vi "PAN_RunProc.vi"(0 "Database RefNum in":T1, 1 "module name":string, 7 "VItoRun":string, 11 "error in (no error)":errorcluster, 12 "wait":bool=TRUE) -> (6 "Result":string, 15 "error out":errorcluster)   [LabVIEW 2016]
uses:
  Modules/DBSHAND/private/vis/DatabaseHand_RefNum.ctl
  <vilib>/Utility/error.llb/DialogType.ctl
  Modules/DBSHAND/private/vis/DatabaseHand_Element_Get(string).vi
panel:
  in  "type specifier VI Refnum (for type only)":refnum<vi>
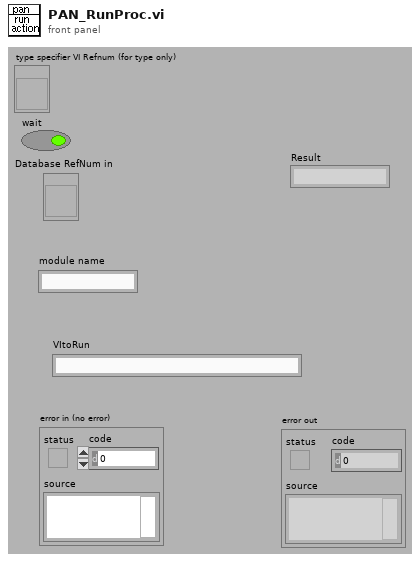
[diagram p1: front panel]
types:
  T1 = typedef "DatabaseHand_RefNum.ctl" = refnum<vi>
  T2 = typedef "DialogType.ctl" = u16
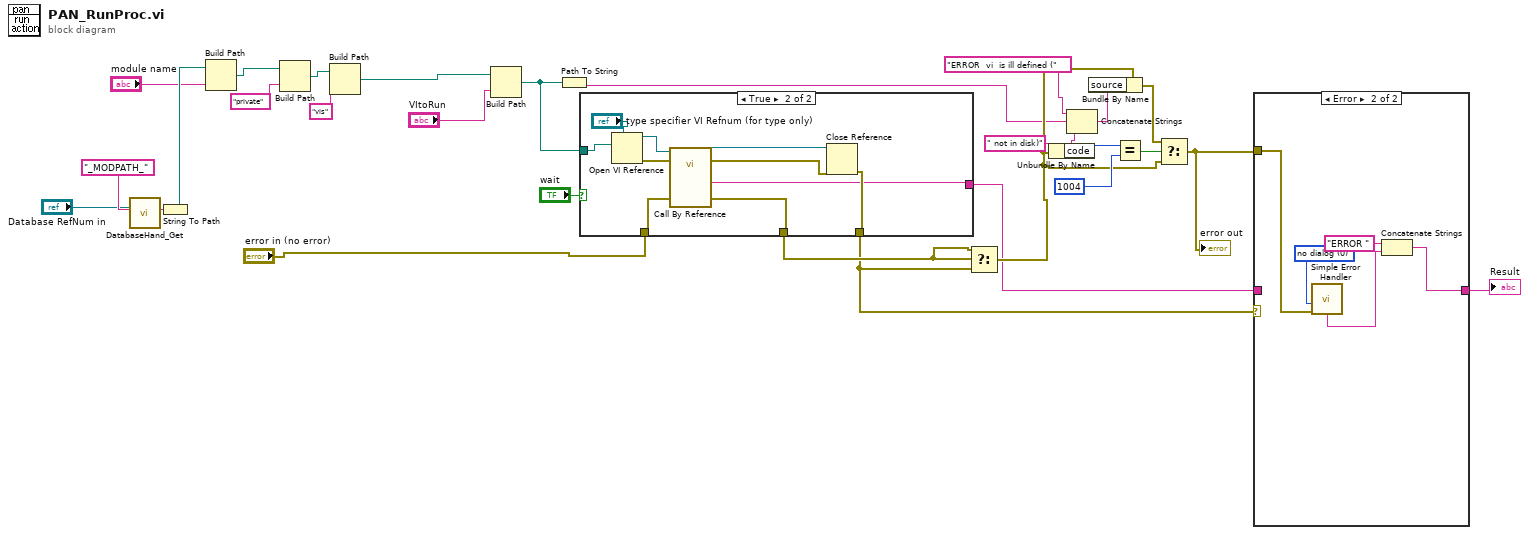
[diagram p0: block diagram]
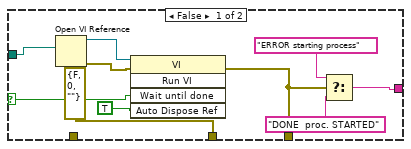
[diagram p3: hidden frame]
diagram:
  n1 = call-poly "DatabaseHand_Get.vi"("name"="_MODPATH_" ("group"), "Database RefNum in"="Database RefNum in") -> ("value"=w14:string)  [unwired: 3 in, 6 out]
  n2 = String To Path(string=w14) -> (path=w13:path)
  n3 = Build Path(base path=w13, name or relative path="module name") -> (appended path=w11:path)
  n4 = Build Path(base path=w11, name or relative path="private") -> (appended path=w9:path)
  n5 = Build Path(base path=w9, name or relative path="vis") -> (appended path=w7:path)
  n6 = Build Path(base path=w7, name or relative path="VItoRun") -> (appended path=w5:path)
  n7 = Path To String(path=w5) -> (string=w4:string)
  n8 = case shown="True" "wait" {
    selector: "wait" -> [w38 _]
    tunnel: [w36 w48] -> w2
    tunnel: "error in (no error)" -> [_ w47]
    tunnel: [errorcluster {"status"=FALSE, "code"=0, "source"=""} ("error out") w46] -> w22
    tunnel: [w33 w43] -> w21
    tunnel: w5 -> [w29 w39]
    frame False {
      n9 = Open VI Reference(vi path=w29) -> (vi reference=w32:refnum<vi>, error out=w31:errorcluster)  [unwired: 2 in, 3 out]
      n10 = invoke class="VI" method="Run VI"(reference=w32, error in=w31, "Wait until done"=w38, "Auto Dispose Ref"=TRUE ("Auto Dispose Reference")) -> (error out=w36:errorcluster)  [unwired: 1 in, 4 out]
      n11 = Select(t="ERROR starting process", s=w36, f="DONE  proc. STARTED" ("Message")) -> (s? t:f=w33:string)
    }
    frame True {
      n12 = Open VI Reference(type specifier VI Refnum (for type only)="type specifier VI Refnum (for type only)", vi path=w39) -> (vi reference=w41:refnum<vi>, error out=w42:errorcluster)  [unwired: 2 in, 2 out]
      n13 = call-by-ref "?"(reference=w41, error in=w42, "error in"=w47) -> (reference out=w44:refnum<vi>, error out=w45:errorcluster, 0:"error out"=w46:errorcluster, "response"=w43:string)  [unwired: 9 in]
      n14 = Close Reference(reference=w44, error in (no error)=w45) -> (error out=w48:errorcluster)
    }
  }
  n15 = Select(t=w22, s=w22, f=w2) -> (s? t:f=w25:errorcluster)
  n16 = Unbundle By Name(w25) -> ("code"=w28:i32)
  n17 = Concatenate Strings("ERROR  vi  is ill defined (" ("source"), w4, " not in disk)") -> (w17:string)
  n18 = Bundle By Name(cluster=w25, "source"=w17) -> (w24:errorcluster)
  n19 = Equal?(x=w28, y=1004) -> (x = y?=w26:bool)
  n20 = Select(t=w24, s=w26, f=w25) -> (s? t:f=w1:errorcluster)
  "error out" <- w1
  n21 = case shown="Error" w2 {
    tunnel: w21 -> [w49 _]
    tunnel: [w49 w51] -> w20
    tunnel: w1 -> [_ w50]
    frame No Error {
    }
    frame Error {
      w54 = T2 0 items=["no dialog", "OK message", "continue or stop message", "OK message + warnings", "continue/stop + warnings"] ("type of dialog (OK msg:1)")
      n22 = call <vilib>:"Simple Error Handler.vi"("type of dialog (OK msg:1)"=w54, "error in (no error)"=w50) -> ("message"=w52:string)  [unwired: 7 out]
      n23 = Concatenate Strings("ERROR " ("string"), w52) -> (w51:string)
    }
  }
  "Result" <- w20
